vi "is a.vi"(8 "error in (no error)":errorcluster, 11 "Thermal Chamber in":refnum<class "Thermal Chamber.lvclass">) -> (0 "error out":errorcluster, 2 "is a":string, 3 "Thermal Chamber out":refnum<class "Thermal Chamber.lvclass">)   [LabVIEW 2016, in "Hardware.lvlib" / "Thermal Chamber.lvclass"]
uses:
  Thermal Chamber.lvclass
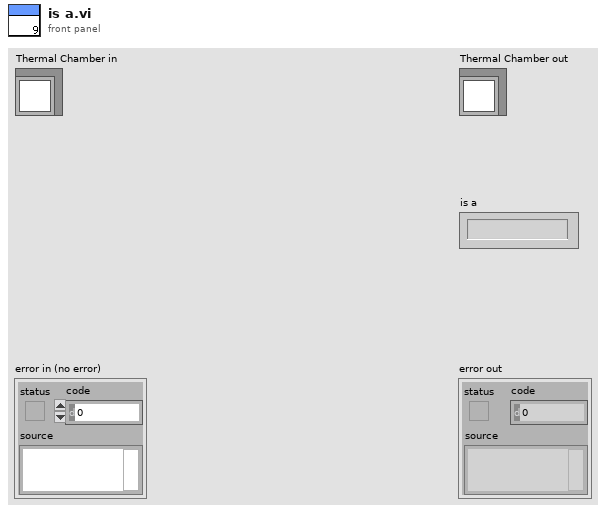
[diagram p1: front panel]
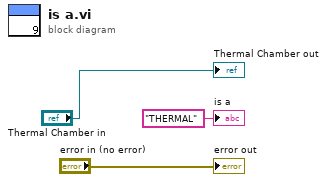
[diagram p0: block diagram]
diagram:
  "error out" <- "error in (no error)"
  "Thermal Chamber out" <- "Thermal Chamber in"
  "is a" <- "THERMAL" ("is a")
